vi "calibrate_kinematics.vi"() -> ()   [LabVIEW 2013]
uses:
  <vilib>/gmath/NI_Gmath.lvlib
  initialization/micron_globals.vi
  <vilib>/Platform/TimedLoop/XDataNode/XDataNode.xnode
  <vilib>/Platform/TimedLoop/XDataNode/nitl_modes.ctl
  <vilib>/Platform/TimedLoop/XDataNode/XDNodeRunTimeDep.lvlib
  <vilib>/Platform/TimedLoop/XDataNode/wakeup.ctl
  <vilib>/Platform/TimedLoop/XDataNode/timing_clust.ctl
  testing/injection_point.ctl
  <vilib>/Analysis/Matrix/Datatypes/RealMatrix.ctl
  <vilib>/Analysis/Matrix/NI_Matrix.lvlib
  testing/probe_point.ctl
  <vilib>/Analysis/Matrix/Numeric/Conversions/Array To Matrix - RA.vi
panel:
  out "Pivot offset":sgl=-11630.0
  out "New tip light positions":T1 format="%#_3f"
  out "Tip light positions":T1 format="%#_3f"
  out "Current handle transform":T1 format="%#_4f"
  out "Tip offset":T1=[[0.0, 0.0, 36200.0]] format="%#.0f"
  in  "Travel scale":sgl=0.5
  out "Handle transform":T1 format="%#_4f"
  out "RMS handle error (microns)":dbl format="%#.2g"
  out "Handle error":T1(graph)
  out "Reconstructed stack motion":dbl[][](graph)
  out "Handle coords output":dbl[][](graph)
  out "Current Kinematics":T1 format="%#_3f"
  out "RMS stack error (microns)":dbl format="%#.2g"
  in  "Store calibration":bool
  out "Inverse kinematics":T1 format="%#_3f"
  in  "Decimate":i32=20
  in  "stop":bool
  in  "Start calibration":bool
  in  "Timescale":i32=500
  # "Inverse kinematics"
  # "Handle transform"
  # "Light positions"
  # "Current value"
  # "New value"
  # "RMS error"
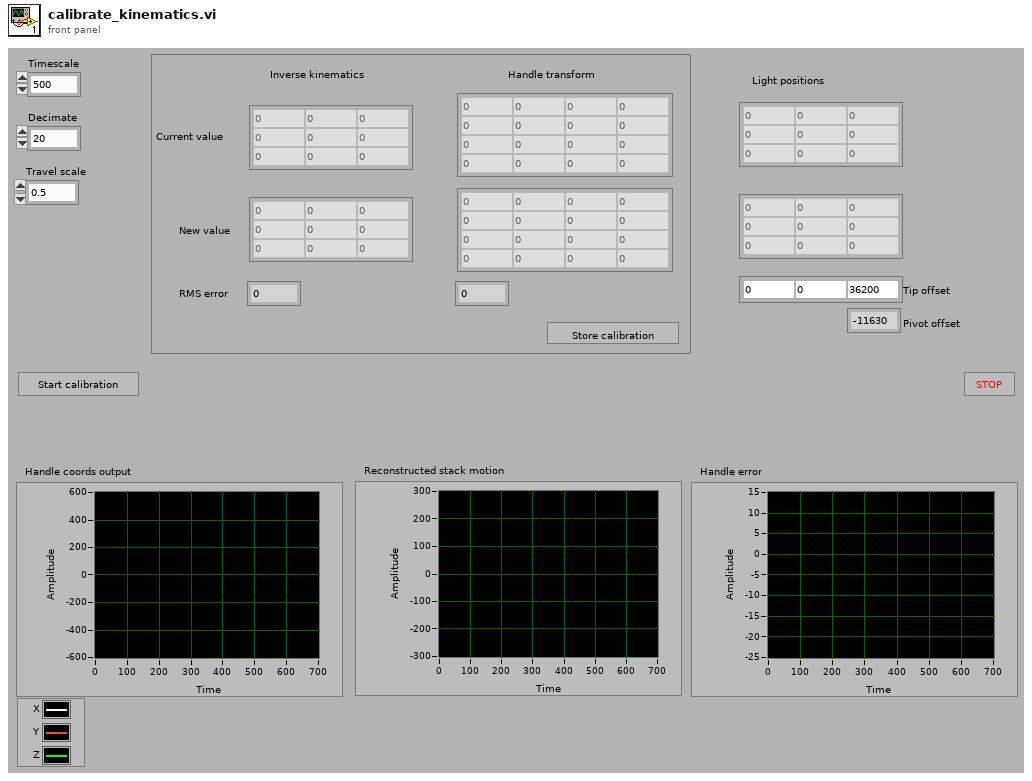
[diagram p1: front panel]
types:
  T1 = typedef "NI_Matrix.lvlib/RealMatrix.ctl" = dbl[][]
  T2 = typedef "injection_point.ctl" = enum16{"Total pose", "V limiter", "Goal ", "Link position", "KF link position", "Inverse kin", "Link goal", "Link error", "Controller", "Output", "Drive", "Light"}
  T3 = enum16{"Off", "Step", "Sine", "Triangle", "Arbitrary"}
  T4 = typedef "probe_point.ctl" = enum16{"Position (tip)", "Position (RCM)", "Null pos (tip)", "Null pos (RCM)", "V limiter (tip)", "V Limiter (RCM)", "Goal (tip)", "Goal (RCM)", "Link pos 0", "Link pos 1", "KF link pos 0", "KF link pos 1", "Link rate 0", "Link rate 1", "Link residue 0", "Link residue 1", "Link goal 0", "Link goal 1", "Rate limit 0", "Rate limit 1", "Link error 0", "Link error 1", "Controller 0", "Controller 1", "Output 0", "Output 1", "Drive 0", "Drive 1", "Stimulus 0", "Stimulus 1", "Trace data 0", "Trace data 1", "Analog data 0", "Analog data 1", "Status flags", "Light 0", "Light 1", "Light 2", "Light 3", "Light 4", "Light 5", "Goal origin", "Goal rotation 0", "Goal rotation 1", "Goal rotation 2", "Output origin", "Output rotation 0", "Output rotation 1", "Output rotation 2", "Handle origin", "Handle rotation 0", "Handle rotation 1", "Handle rotation 2", "Handle position", "Handle velocity", "Handle acceleration", "Handle angles", "Handle angle rates", "Handle pos residue", "Handle angle residue", "Trace length"}
  T5 = typedef "XDNodeRunTimeDep.lvlib/timing_clust.ctl" = cluster{"Expected End [f-1]":u64, "Actual End [f-1]":u64, "Finished Late? [f-1]":bool, "Expected End [i-1]":u64, "Actual End [i-1]":u64, "Finished Late? [i-1]":bool, "Expected Start [i]":u64, "Actual Start [i]":u64, "Expected Start [f]":u64, "Actual Start [f]":u64, "Source Name":string, "Structure Name":string, "Period":i64, "Deadline":i64, "Offset":i64, "Start":i64, "Priority":i32, "Timeout":i32, "Mode":T6, "Wakeup Reason":T7, "Error":errorcluster, "Source Type":string, "Secondary Source Type":string, "Global End Time":u64, "Global Start Time":u64, "Frame Duration":u64, "Iteration Duration":u64, "Assigned CPU":i32, "I/O Scan Engine Mode":u32}
  T6 = typedef "XDNodeRunTimeDep.lvlib/nitl_modes.ctl" = enum32{"No Change", "Process missed periods, maintain original phase", "Discard missed periods, maintain original phase", "Process missed periods, ignore original phase", "Discard missed periods, ignore original phase"}
  T7 = typedef "XDNodeRunTimeDep.lvlib/wakeup.ctl" = enum32{"Normal", "Aborted", "Asynchronous wakeup", "Timing source error", "Timed loop error", "Timeout"}
  T8 = typedef "Micron params.ctl" = cluster{"Stimulus":T9, "Goal Filter A":T10, "Mode controls":T11, "Manipulator type":enum16{"Current piezo", "Voltage piezo"}, "Manipulator calibration":T12, "Network":T14, "Goal Filter B":T10, "Cancellation":T15, "Transition time":sgl, "Estimation":T17}
  T9 = typedef "stimulus.ctl" = cluster{"Type":enum16{"Off", "Step", "Sine", "Triangle", "Arbitrary"}, "Phase":dbl, "Amplitude":sgl[], "Injection point":T2, "Closed loop":bool, "Offset":sgl[], "Tip -> world":bool, "Frequency":dbl, "Length":dbl}
  T10 = typedef "goal_loop_parms.ctl" = cluster{"Speedup max":sgl, "Speedup thresh":sgl, "Speedup nonlin":sgl, "Filters":cluster{"Lower Fc":sgl, "Lower Q":sgl, "Scale factor":sgl, "Upper Fc":sgl, "Upper Q":sgl, "V limit":sgl, "V limit range":sgl}[]}
  T11 = typedef "mode_conrols.ctl" = cluster{"Hold":bool, "Cancellation":bool, "Goal filter":bool, "Trigger":bool}
  T12 = typedef "manipulator_cal.ctl" = cluster{"Tool offsets":sgl[][], "Tip light calibration":T13, "Handle light calibration":T13, "Base pivots":sgl[][], "Output pivots":sgl[][], "Length center":sgl, "Workspace height":sgl[], "Workspace diameter":sgl[], "Linearization":sgl[][], "Stack travel":sgl, "Saturation pos":sgl, "Inverse filters":cluster{"filter structure":enum32{"IIR 2nd Order", "IIR 4th Order"}, "Reverse Coefficients":dbl[], "Forward Coefficients":dbl[]}[]}
  T13 = typedef "probe_calibration.ctl" = sgl[][]
  T14 = typedef "network_params.ctl" = cluster{"Remote Host":string, "Send Status":bool, "Send Port":u16, "Recv Commands":bool, "Recv Port":u16}
  T15 = typedef "sq_control_params.ctl" = cluster{"KP":T16, "KI":sgl, "KD":T16, "Max vel":sgl, "Max acc":sgl, "Int error limit":sgl, "RCM gain":sgl, "Bypass":bool, "Degraded gain":sgl}
  T16 = typedef "decoupled_gain.ctl" = cluster{"XY":sgl, "Rxy":sgl, "Z":sgl, "Rz":sgl}
  T17 = typedef "estimation_controls.ctl" = cluster{"Link":cluster{"Measure noise":dbl[], "Process noise":dbl[], "Alt process noise":dbl[], "Alt turnoff cycles":i32, "Innovation limit":dbl[], "Residue threshold":dbl, "Enable":bool}, "Handle":cluster{"Measure noise":dbl[], "Process noise":dbl[], "State limits":dbl[], "Innovation limit":dbl[], "Prediction Lookahead":sgl, "Enable":bool}}
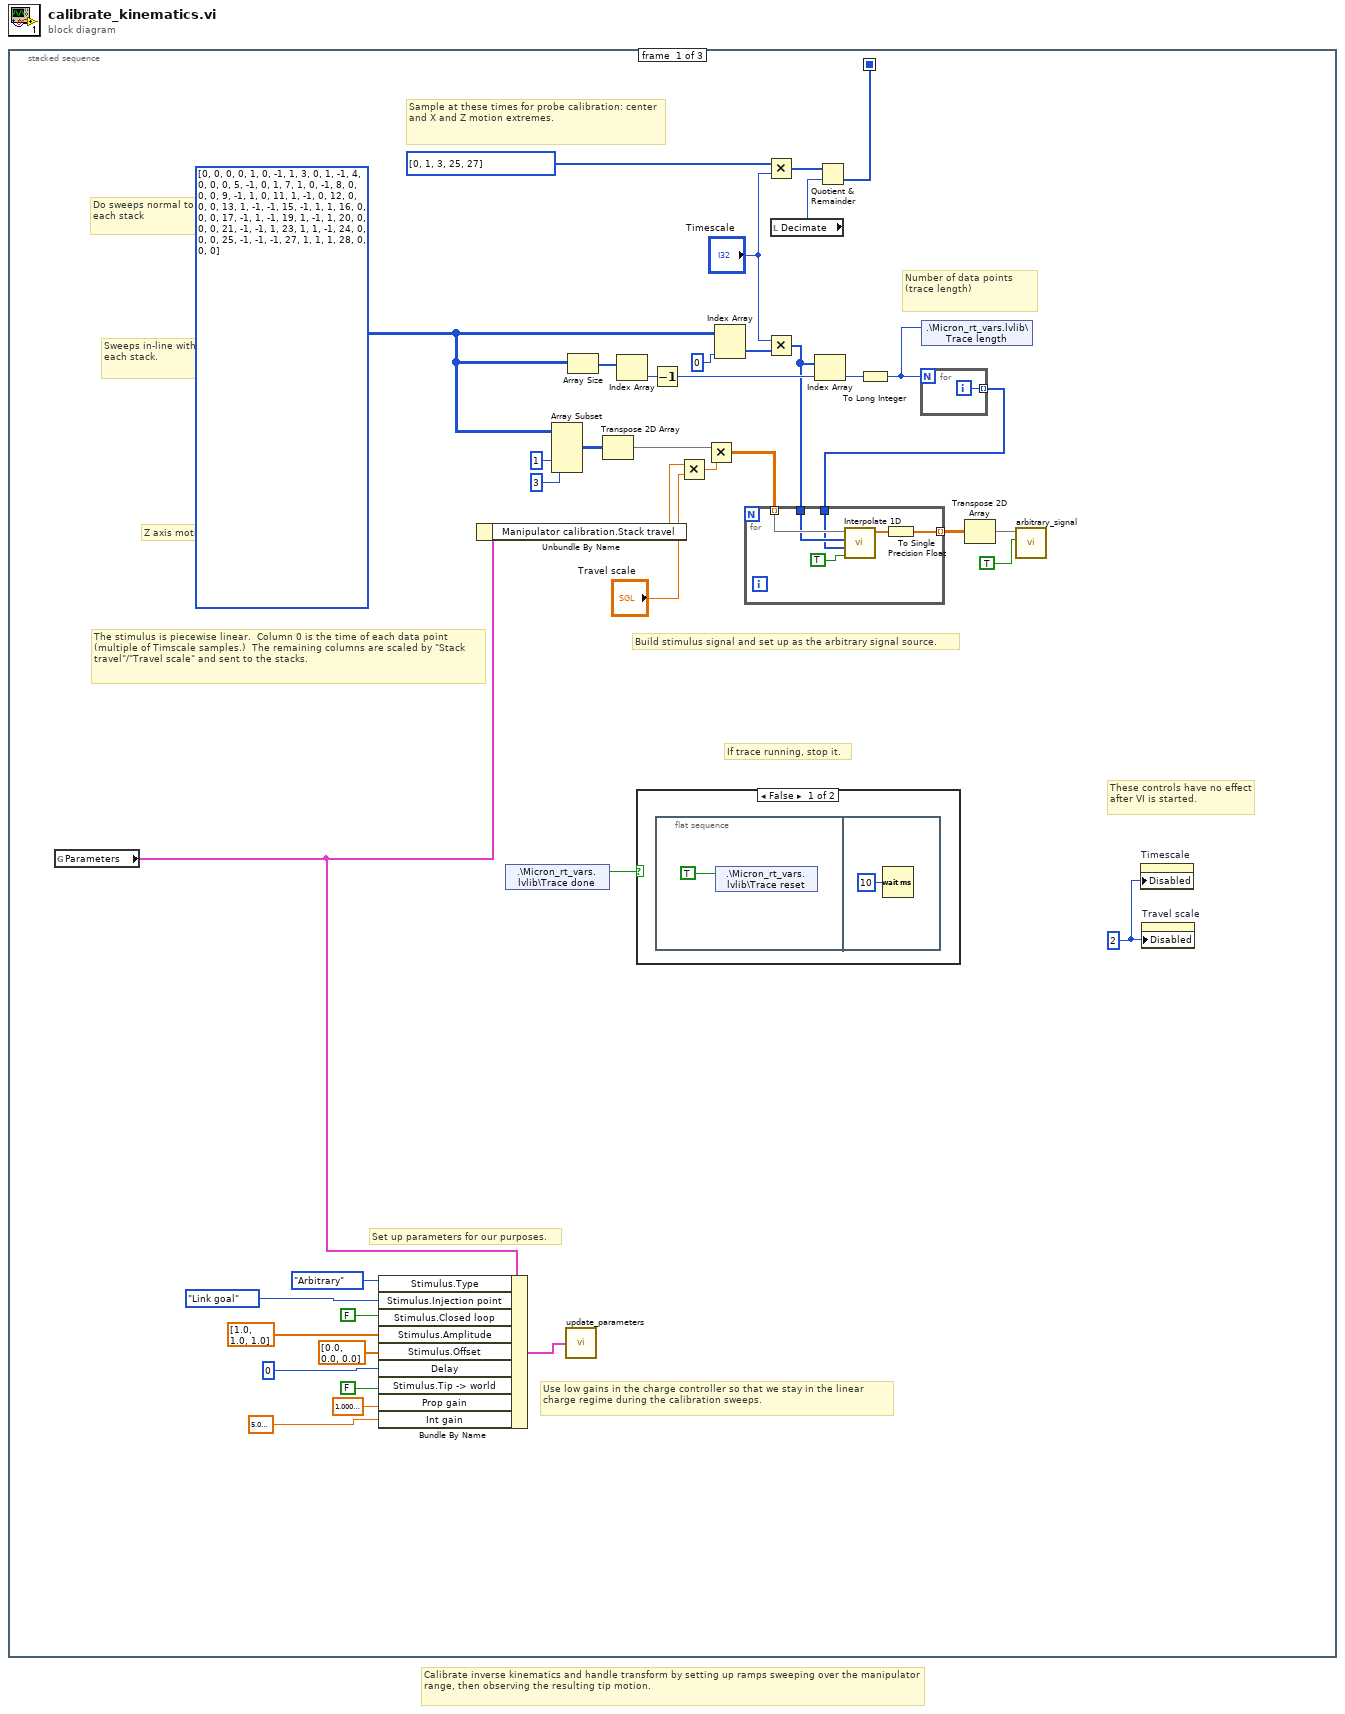
[diagram p0: block diagram]
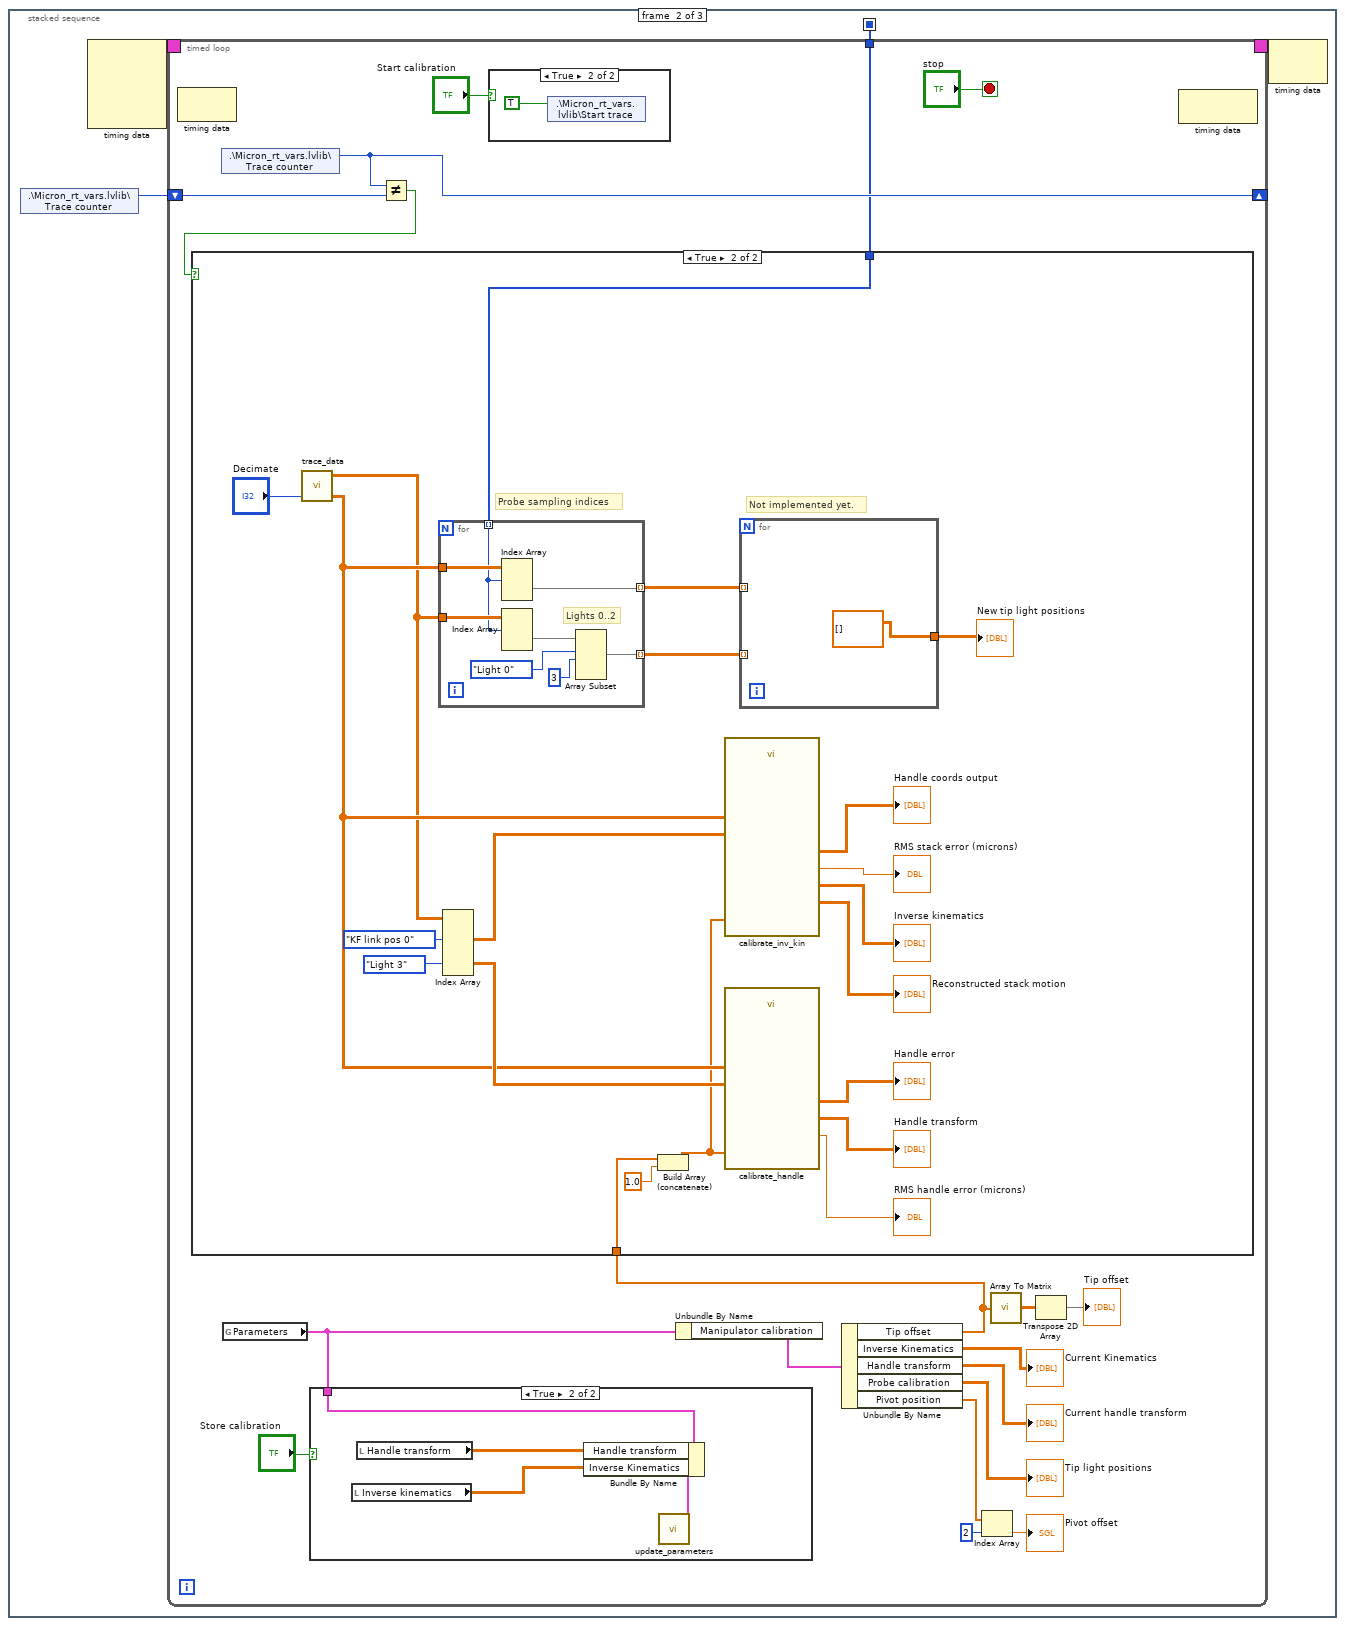
[diagram p3: hidden frame]
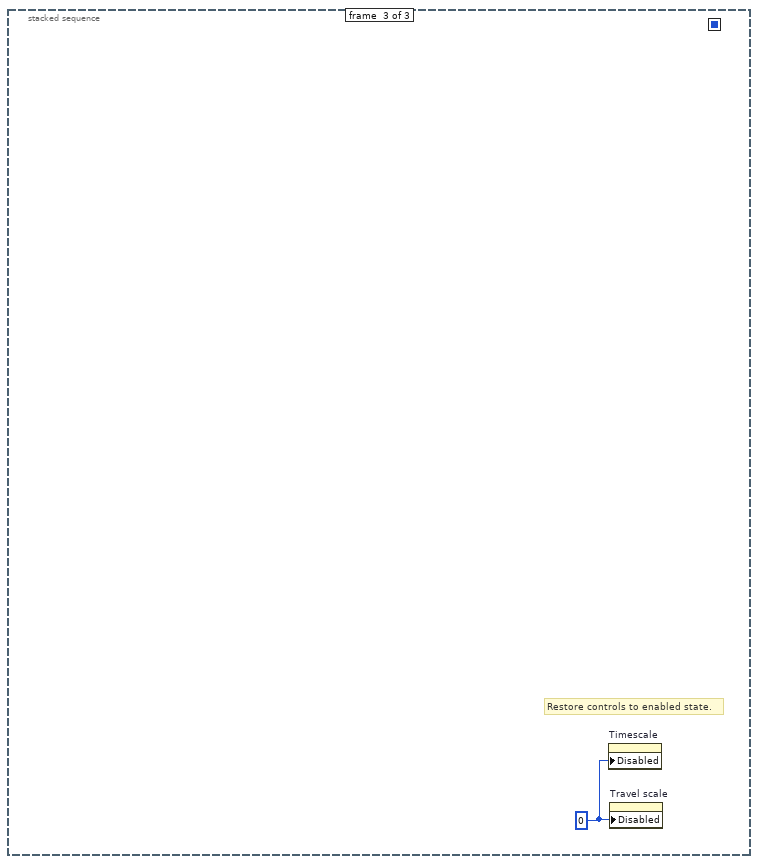
[diagram p7: hidden frame]
diagram:
  # "Calibrate inverse kinematics and handle transform by setting up ramps sweeping over the manipulator range, then observing the resulting tip motion."
  n1 = stacked-sequence {
    seq-local: [w8 _ _] -> [_ w49 _]
    frame #0 {
      w14 = u8 2 ("Disabled")
      w33 = i32[][] [[0, 0, 0, 0], [1, 0, -1, 1], [3, 0, 1, -1], [4, 0, 0, 0], [5, -1, 0, 1], [7, 1, 0, -1], [8, 0, 0, 0], [9, -1, 1, 0], [11, 1, -1, 0], [12, 0, 0, 0], [13, 1, -1, -1], [15, -1, 1, 1], [16, 0, 0, 0], [17, -1, 1, -1], [19, 1, -1, 1], [20, 0, 0, 0], [21, -1, -1, 1], [23, 1, 1, -1], [24, 0, 0, 0], [25, -1, -1, -1], [27, 1, 1, 1], [28, 0, 0, 0]]
      # "Use low gains in the charge controller so that we stay in the linear charge regime during the calibration sweeps."
      # "Sample at these times for probe calibration: center and X and Z motion extremes."
      # "The stimulus is piecewise linear.  Column 0 is the time of each data point (multiple of Timscale samples.)  The remaining columns are scaled by \"Stack travel\"/\"Travel scale\" and sent to the stacks."
      # "Build stimulus signal and set up as the arbitrary signal source."
      # "Set up parameters for our purposes."
      # "These controls have no effect after VI is started."
      # "If trace running, stop it."
      # "Number of data points (trace length)"
      # "Z axis motion"
      # "Sweeps in-line with each stack."
      # "Do sweeps normal to each stack"
      n2 = global read "micron_globals.vi" "Parameters"() -> (w5:T8)
      n3 = Bundle By Name(cluster=w5, "Stimulus.Type"=T3."Arbitrary" ("Type"), "Stimulus.Injection point"=injection_point."Link goal" ("Injection point"), "Stimulus.Closed loop"=FALSE ("Closed loop"), "Stimulus.Amplitude"=sgl[] [1.0, 1.0, 1.0] ("Amplitude"), "Stimulus.Offset"=sgl[] [0.0, 0.0, 0.0] ("Amplitude"), "Delay"=0, "Stimulus.Tip -> world"=FALSE, "Prop gain"=sgl 1e-07 ("Charge piezo.Prop gain"), "Int gain"=sgl 5e-11 ("Charge piezo.Prop gain")) -> (w6:T8)
      n4 = Unbundle By Name(w5) -> ("Manipulator calibration.Stack travel"=w4:sgl)
      n5 = shared-variable ".\\Micron_rt_vars.lvlib\\Trace done"() -> (w13:bool)  [unwired: 2 out]
      n6 = Array Subset(array=w33, index (col)=1 ("index"), length (col)=3 ("length")) -> (w30:i32[][])  [unwired: 2 in]
      n7 = call "update_parameters.vi"("Parameters"=w6) -> ()
      n8 = Array Size(array=w33) -> (size(s)=w38:i32[])
      n9 = Transpose 2D Array(2D array=w30) -> (transposed array=w17:i32[][])
      n10 = Index Array(array=w38) -> (element=w37:i32)  [unwired: 1 in]
      n11 = case shown="False" w13 {
        frame False {
          n12 = flat-sequence {
            frame #0 {
              n13 = shared-variable ".\\Micron_rt_vars.lvlib\\Trace reset"(TRUE ("Start trace")) -> ()  [unwired: 2 out]
            }
            frame #1 {
              n14 = Wait (ms)(milliseconds to wait=u32 10) -> ()  [unwired: 1 out]
            }
          }
        }
        frame True {
        }
      }
      n15 = Decrement(x=w37) -> (x-1=w34:i32)
      n16 = Multiply(x=w4, y="Travel scale") -> (x*y=w16:sgl)
      n17 = Multiply(x=w17, y=w16) -> (x*y=w18:sgl[][])
      n18 = Index Array(array=w33, index (col)=0 ("disabled index (col)")) -> (element=w35:i32[])  [unwired: 1 in]
      n19 = Multiply(x=i32[] [0, 1, 3, 25, 27], y="Timescale") -> (x*y=w11:i32[])
      n20 = Multiply(x="Timescale", y=w35) -> (x*y=w28:i32[])
      n21 = local read "Decimate"() -> (w10:i32)
      n22 = Index Array(array=w28, index=w34) -> (element=w24:i32)
      n23 = Quotient & Remainder(x=w11, y=w10) -> (floor(x/y)=w8:i32[])  [unwired: 1 out]
      n24 = To Long Integer(number=w24) -> (32bit integer=w7:i32)
      n25 = for {
        N: w7 -> [_]
        tunnel: [w42] -> w29 mode=indexing
        i -> [w42]
      }
      n26 = for {
        tunnel: w18 -> [w48] mode=indexing
        tunnel: w29 -> [w46]
        tunnel: w28 -> [w47]
        tunnel: [w43] -> w26 mode=indexing
        n27 = call <vilib>:"Interpolate 1D.vi"("X is monotonic"=TRUE, "xi"=w46, "X"=w47, "Y"=w48) -> ("yi"=w44:dbl[])  [unwired: 2 in, 5 out]
        n28 = To Single Precision Float(number=w44) -> (single precision float=w43:sgl[])
      }
      n29 = shared-variable ".\\Micron_rt_vars.lvlib\\Trace length"(w7) -> ()  [unwired: 2 out]
      n30 = Transpose 2D Array(2D array=w26) -> (transposed array=w25:sgl[][])
      n31 = call "arbitrary_signal.vi"("Set signal"=TRUE, "New signal"=w25) -> ()  [unwired: 1 in, 9 out]
      n32 = property on="Timescale" class="DigNum (strict)"("Disabled"=w14) -> ()  [unwired: 2 in, 2 out]
      n33 = property on="Travel scale" class="DigNum (strict)"("Disabled"=w14) -> ()  [unwired: 2 in, 2 out]
    }
    frame #1 {
      n34 = shared-variable ".\\Micron_rt_vars.lvlib\\Trace counter"() -> (w50:u32)  [unwired: 2 out]
      n35 = node-c288() -> (w52:T5)  [unwired: 4 out]
      n36 = timed-loop {
        timing: w52 -> [_]
        timing-out: [_] -> w51
        shift-right: [w68] -> _
        shift-left: w50 -> [w69]
        tunnel: w49 -> [w64]
        stop <- "stop" stop-if-true
        n37 = node-c288() -> ()  [unwired: 2 out]
        n38 = shared-variable ".\\Micron_rt_vars.lvlib\\Trace counter"() -> (w68:u32)  [unwired: 2 out]
        n39 = global read "micron_globals.vi" "Parameters"() -> (w54:T8)
        n40 = case shown="True" "Store calibration" {
          tunnel: w54 -> [_ w72]
          frame False {
          }
          frame True {
            n41 = local read "Inverse kinematics"() -> (w73:T1)
            n42 = local read "Handle transform"() -> (w74:T1)
            n43 = Bundle By Name(cluster=w72, "Handle transform"=w74, "Inverse Kinematics"=w73) -> (w71:T8)
            n44 = call "update_parameters.vi"("Parameters"=w71) -> ()
          }
        }
        n45 = Not Equal?(x=w68, y=w69) -> (x != y?=w67:bool)
        n46 = case shown="True" "Start calibration" {
          frame False {
          }
          frame True {
            n47 = shared-variable ".\\Micron_rt_vars.lvlib\\Start trace"(TRUE ("Start trace")) -> ()  [unwired: 2 out]
          }
        }
        n48 = Unbundle By Name(w54) -> ("Manipulator calibration"=w57:T12)
        n49 = Unbundle By Name(w57) -> ("Tip offset"=w53:sgl[], "Inverse Kinematics"=→"Current Kinematics":T1, "Handle transform"=→"Current handle transform":T1, "Probe calibration"=→"Tip light positions":T13, "Pivot position"=w59:sgl[])
        n50 = case shown="True" w67 {
          tunnel: w64 -> [_ w85]
          tunnel: w53 -> [_ w77]
          frame False {
          }
          frame True {
            # "Not implemented yet."
            # "Probe sampling indices"
            n51 = call "trace_data.vi"("Decimate"="Decimate") -> ("Decimated pose (manipulator)"=w86:dbl[][][], "Decimated trace"=w84:sgl[][][])  [unwired: 2 in, 1 out]
            n52 = for {
              tunnel: w86 -> [w104]
              tunnel: w85 -> [w101] mode=indexing
              tunnel: w84 -> [w102]
              tunnel: [w99] -> w83 mode=indexing
              tunnel: [w98] -> w82 mode=indexing
              # "Lights 0..2"
              n53 = Index Array(array=w104, index (dim 0)=w101) -> (element=w99:dbl[][])  [unwired: 2 in]
              n54 = Index Array(array=w102, index (dim 0)=w101) -> (element=w100:sgl[][])  [unwired: 2 in]
              n55 = Array Subset(array=w100, index (row)=probe_point."Light 0" ("Probe point"), length (row)=3 ("length")) -> (w98:sgl[][])  [unwired: 2 in]
            }
            n56 = Index Array(array=w84, index (dim 1) #1=probe_point."KF link pos 0" ("Probe point"), index (dim 1) #2=probe_point."Light 3" ("Probe point")) -> (element #1=w91:sgl[][], element #2=w90:sgl[][])  [unwired: 4 in]
            n57 = Build Array (concatenate)(w77, sgl 1.0 ("Numeric")) -> (w75:sgl[])
            n58 = call "calibrate_inv_kin.vi"("Stimulus"=w91, "Decimated pose (manipulator)"=w86, "Tip offset"=w75) -> ("Calibrated"=→"Reconstructed stack motion":T1, "Error"=→"RMS stack error (microns)":dbl, "New kinematics"=→"Inverse kinematics":T1, "Handle coords output"=→"Handle coords output":dbl[][])  [unwired: 5 out]
            n59 = call "calibrate_handle.vi"("Decimated pose (manipulator)"=w86, "Tip offset"=w75, "Light 3 pos"=w90) -> ("Handle error"=→"Handle error":T1, "RMS Error"=→"RMS handle error (microns)":dbl, "Handle transform"=→"Handle transform":T1)  [unwired: 6 out]
            n60 = for {
              tunnel: w83 -> [_] mode=indexing
              tunnel: w82 -> [_] mode=indexing
              tunnel: [T1 [] ("New tip light positions")] -> w81
            }
            "New tip light positions" <- w81
          }
        }
        n61 = Index Array(array=w59, index=2) -> (element=→"Pivot offset":sgl)
        n62 = call-poly <vilib>:"Array To Matrix.vi"("Real 1D Array"=w53) -> ("Real Matrix (Column Vector)"=w56:T1)
        n63 = Transpose 2D Array(2D array=w56) -> (transposed array=→"Tip offset":T1)
        n64 = node-c288() -> ()  [unwired: 2 out]
      }
      n65 = node-c288(w51) -> ()  [unwired: 1 out]
    }
    frame #2 {
      w110 = u8 0 ("Disabled")
      # "Restore controls to enabled state."
      n66 = property on="Timescale" class="DigNum (strict)"("Disabled"=w110) -> ()  [unwired: 2 in, 2 out]
      n67 = property on="Travel scale" class="DigNum (strict)"("Disabled"=w110) -> ()  [unwired: 2 in, 2 out]
    }
  }
